vi "Analysis-SD-Core.vi"(11 "all rows":dbl[][](array[numeric])) -> (1 "variance":dbl format="%0.6f", 2 "standard deviation":dbl format="%0.6f", 3 "mean":dbl format="%0.4f", 4 "XY Graph":T1(graph), 5 "média erro %":dbl format="%0.6f", 6 "média SD":dbl format="%0.6f")   [LabVIEW 2014]
uses:
  <vilib>/Analysis/NI_AALBase.lvlib
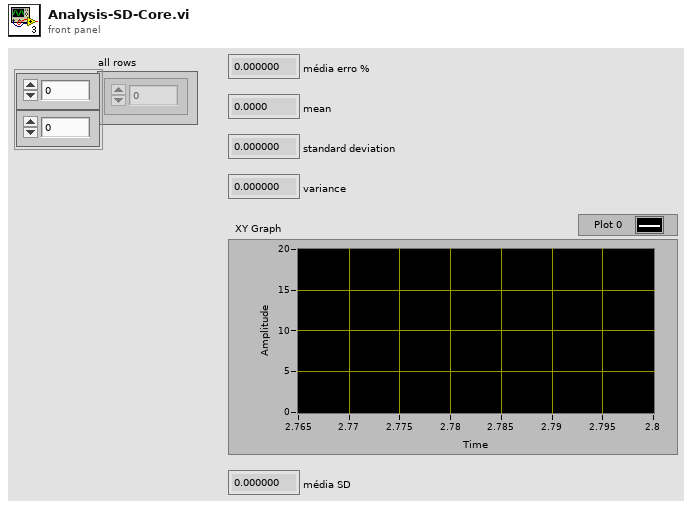
[diagram p1: front panel]
types:
  T1 = cluster{"X Values":dbl[], "Histogram: h(x)":i32[]}
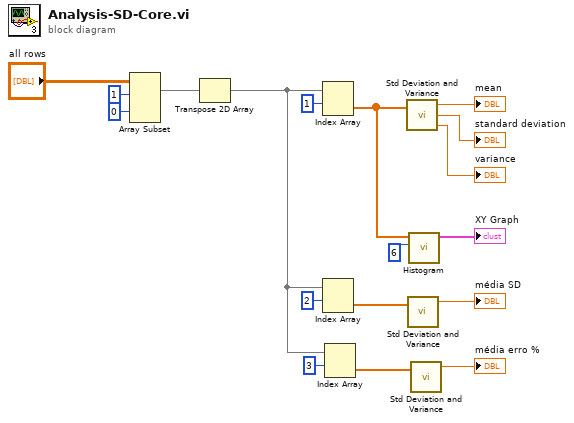
[diagram p0: block diagram]
diagram:
  n1 = Array Subset(array="all rows", index (row)=1 ("index"), index (col)=0 ("index")) -> (w6:dbl[][])  [unwired: 2 in]
  n2 = Transpose 2D Array(2D array=w6) -> (transposed array=w16:dbl[][])
  n3 = Index Array(array=w16, index (row)=1) -> (element=w7:dbl[])  [unwired: 1 in]
  n4 = Index Array(array=w16, index (row)=2) -> (element=w13:dbl[])  [unwired: 1 in]
  n5 = Index Array(array=w16, index (row)=3) -> (element=w17:dbl[])  [unwired: 1 in]
  n6 = call <vilib>:"Std Deviation and Variance.vi"("X"=w7) -> ("mean"=→"mean":dbl, "standard deviation"=→"standard deviation":dbl, "variance"=→"variance":dbl)  [unwired: 1 in]
  n7 = call <vilib>:"Std Deviation and Variance.vi"("X"=w13) -> ("mean"=→"média SD":dbl)  [unwired: 1 in, 2 out]
  n8 = call <vilib>:"Histogram.vi"("intervals"=6, "X"=w7) -> ("Histogram Graph"=→"XY Graph":T1)  [unwired: 6 in, 3 out]
  n9 = call <vilib>:"Std Deviation and Variance.vi"("X"=w17) -> ("mean"=→"média erro %":dbl)  [unwired: 1 in, 2 out]
